vi "S4GUI.vi"(7 "Tab ObsEng":enum32{"Obs", "CCD modes", "Guider", "Eng"}(tab)) -> ()   [LabVIEW 2018] (continued)
            n3113 = call-dynamic "Write Object.vi"("error in (no error)"=w6663, "Object"=w6746, "Interface in"=w6666) -> ("error out"=w6664:errorcluster, "Interface out"=w6667:refnum<class "Interface.lvclass">)  [unwired: 7 in]
            n3114 = call-dynamic "Write Object.vi"("error in (no error)"=w6559, "Object"=w6746, "Interface in"=w6562) -> ("error out"=w6560:errorcluster, "Interface out"=w6563:refnum<class "Interface.lvclass">)  [unwired: 7 in]
            n3115 = call-dynamic "Write Object.vi"("error in (no error)"=w6618, "Object"=w6746, "Interface in"=w6615) -> ("error out"=w6617:errorcluster, "Interface out"=w6614:refnum<class "Interface.lvclass">)  [unwired: 7 in]
            n3116 = call-dynamic "Write Comments.vi"("error in (no error)"=w6664, "Comments"=w6745, "Interface in"=w6667) -> ("error out"=w6668:errorcluster, "Interface out"=w6669:refnum<class "Interface.lvclass">)  [unwired: 7 in]
            n3117 = call-dynamic "Write Comments.vi"("error in (no error)"=w6713, "Comments"=w6745, "Interface in"=w6717) -> ("error out"=w6718:errorcluster, "Interface out"=w6719:refnum<class "Interface.lvclass">)  [unwired: 7 in]
            n3118 = call-dynamic "Write Comments.vi"("error in (no error)"=w6560, "Comments"=w6745, "Interface in"=w6563) -> ("error out"=w6564:errorcluster, "Interface out"=w6565:refnum<class "Interface.lvclass">)  [unwired: 7 in]
            n3119 = call-dynamic "Write Comments.vi"("error in (no error)"=w6617, "Comments"=w6745, "Interface in"=w6614) -> ("error out"=w6613:errorcluster, "Interface out"=w6612:refnum<class "Interface.lvclass">)  [unwired: 7 in]
            n3120 = call-dynamic "Write Observer.vi"("error in (no error)"=w6668, "Observer"=w6744, "Interface in"=w6669) -> ("error out"=w6673:errorcluster, "Interface out"=w6672:refnum<class "Interface.lvclass">)  [unwired: 7 in]
            n3121 = call-dynamic "Write Observer.vi"("error in (no error)"=w6718, "Observer"=w6744, "Interface in"=w6719) -> ("error out"=w6723:errorcluster, "Interface out"=w6722:refnum<class "Interface.lvclass">)  [unwired: 7 in]
            n3122 = call-dynamic "Write Observer.vi"("error in (no error)"=w6564, "Observer"=w6744, "Interface in"=w6565) -> ("error out"=w6530:errorcluster, "Interface out"=w6531:refnum<class "Interface.lvclass">)  [unwired: 7 in]
            n3123 = call-dynamic "Write Observer.vi"("error in (no error)"=w6613, "Observer"=w6744, "Interface in"=w6612) -> ("error out"=w6608:errorcluster, "Interface out"=w6609:refnum<class "Interface.lvclass">)  [unwired: 7 in]
            n3124 = call-dynamic "Write Interface.vi"("error in (no error)"=w6723, "Interface.lvclass"=w6722, "Channel in"=w6714) -> ("error out"=w6706:errorcluster, "Channel out"=w6707:refnum<class "Channel.lvclass">)  [unwired: 7 in]
            n3125 = call-dynamic "Write Interface.vi"("error in (no error)"=w6608, "Interface.lvclass"=w6609, "Channel in"=w6621) -> ("error out"=w6585:errorcluster, "Channel out"=w6586:refnum<class "Channel.lvclass">)  [unwired: 7 in]
            n3126 = call-dynamic "Write Interface.vi"("error in (no error)"=w6673, "Interface.lvclass"=w6672, "Channel in"=w6659) -> ("error out"=w6637:errorcluster, "Channel out"=w6639:refnum<class "Channel.lvclass">)  [unwired: 7 in]
            n3127 = call-dynamic "Write Interface.vi"("error in (no error)"=w6530, "Interface.lvclass"=w6531, "Channel in"=w6532) -> ("error out"=w6535:errorcluster, "Channel out"=w6536:refnum<class "Channel.lvclass">)  [unwired: 7 in]
            n3128 = case shown="True" w6526 {
              tunnel: [w6874 w6896] -> w6727
              tunnel: [w6873 w6895] -> w6726
              tunnel: w6707 -> [w6874 w6894]
              tunnel: w6706 -> [w6873 w6893]
              frame False {
              }
              frame True {
                n3129 = call-dynamic "Read State Machine.vi"("error in (no error)"=w6893, "Device in"=w6894) -> ("error out"=w6890:errorcluster, "State Machine.lvclass"=w6891:refnum<class "State Machine.lvclass">, "Device out"=w6898:refnum<class "Channel.lvclass">)  [unwired: 7 in]
                n3130 = call-dynamic "Read ref StatesQueue.vi"("error in (no error)"=w6890, "State Machine in"=w6891) -> ("error out"=w6888:errorcluster, "ref StatesQueue"=w6889:refnum<queue>, "State Machine out"=w6885:refnum<class "State Machine.lvclass">)  [unwired: 7 in]
                n3131 = Flush Queue(queue=w6889, error in (no error)=w6888) -> (queue out=w6887:refnum<queue>, error out=w6883:errorcluster)  [unwired: 1 out]
                n3132 = Enqueue Element(queue=w6887, element=u32 300 ("State"), error in (no error)=w6883) -> (queue out=w6878:refnum<queue>, error out=w6876:errorcluster)  [unwired: 1 in, 1 out]
                n3133 = disable-structure shown="Enabled" {
                  disable-tunnel: w6878 -> [w6904 w6906]
                  disable-tunnel: [w6903 w6906] -> w6877
                  disable-tunnel: w6876 -> [w6902 w6905]
                  disable-tunnel: [w6901 w6905] -> w6875
                  frame Disabled {
                    n3134 = Enqueue Element(queue=w6904, element=u32 305 ("State"), error in (no error)=w6902) -> (queue out=w6903:refnum<queue>, error out=w6901:errorcluster)  [unwired: 1 in, 1 out]
                  }
                  frame Enabled {
                  }
                }
                n3135 = Enqueue Element(queue=w6877, element=u32 60 ("State"), error in (no error)=w6875) -> (queue out=w6886:refnum<queue>, error out=w6884:errorcluster)  [unwired: 1 in, 1 out]
                n3136 = call-dynamic "Write ref StatesQueue.vi"("error in (no error)"=w6884, "ref StatesQueue"=w6886, "State Machine in"=w6885) -> ("error out"=w6881:errorcluster, "State Machine out"=w6882:refnum<class "State Machine.lvclass">)  [unwired: 7 in]
                n3137 = call-dynamic "Write State.vi"("error in (no error)"=w6881, "State"=0, "State Machine in"=w6882) -> ("error out"=w6899:errorcluster, "State Machine out"=w6897:refnum<class "State Machine.lvclass">)  [unwired: 7 in]
                n3138 = call-dynamic "Write State Machine.vi"("error in (no error)"=w6899, "State Machine.lvclass"=w6897, "Device in"=w6898) -> ("error out"=w6895:errorcluster, "Device out"=w6896:refnum<class "Channel.lvclass">)  [unwired: 7 in]
              }
            }
            n3139 = case shown="True" w6527 {
              tunnel: w6639 -> [w6840 w6849]
              tunnel: [w6840 w6847] -> w6638
              tunnel: w6637 -> [w6839 w6846]
              tunnel: [w6839 w6845] -> w6636
              frame False {
              }
              frame True {
                n3140 = call-dynamic "Read State Machine.vi"("error in (no error)"=w6846, "Device in"=w6849) -> ("error out"=w6861:errorcluster, "State Machine.lvclass"=w6862:refnum<class "State Machine.lvclass">, "Device out"=w6848:refnum<class "Channel.lvclass">)  [unwired: 7 in]
                n3141 = call-dynamic "Read ref StatesQueue.vi"("error in (no error)"=w6861, "State Machine in"=w6862) -> ("error out"=w6859:errorcluster, "ref StatesQueue"=w6860:refnum<queue>, "State Machine out"=w6856:refnum<class "State Machine.lvclass">)  [unwired: 7 in]
                n3142 = Flush Queue(queue=w6860, error in (no error)=w6859) -> (queue out=w6858:refnum<queue>, error out=w6854:errorcluster)  [unwired: 1 out]
                n3143 = Enqueue Element(queue=w6858, element=u32 300 ("State"), error in (no error)=w6854) -> (queue out=w6844:refnum<queue>, error out=w6842:errorcluster)  [unwired: 1 in, 1 out]
                n3144 = disable-structure shown="Enabled" {
                  disable-tunnel: w6844 -> [w6869 w6872]
                  disable-tunnel: [w6868 w6872] -> w6843
                  disable-tunnel: w6842 -> [w6867 w6871]
                  disable-tunnel: [w6866 w6871] -> w6841
                  frame Disabled {
                    n3145 = Enqueue Element(queue=w6869, element=u32 305 ("State"), error in (no error)=w6867) -> (queue out=w6868:refnum<queue>, error out=w6866:errorcluster)  [unwired: 1 in, 1 out]
                  }
                  frame Enabled {
                  }
                }
                n3146 = Enqueue Element(queue=w6843, element=u32 60 ("State"), error in (no error)=w6841) -> (queue out=w6857:refnum<queue>, error out=w6855:errorcluster)  [unwired: 1 in, 1 out]
                n3147 = call-dynamic "Write ref StatesQueue.vi"("error in (no error)"=w6855, "ref StatesQueue"=w6857, "State Machine in"=w6856) -> ("error out"=w6852:errorcluster, "State Machine out"=w6853:refnum<class "State Machine.lvclass">)  [unwired: 7 in]
                n3148 = call-dynamic "Write State.vi"("error in (no error)"=w6852, "State"=0, "State Machine in"=w6853) -> ("error out"=w6865:errorcluster, "State Machine out"=w6864:refnum<class "State Machine.lvclass">)  [unwired: 7 in]
                n3149 = call-dynamic "Write State Machine.vi"("error in (no error)"=w6865, "State Machine.lvclass"=w6864, "Device in"=w6848) -> ("error out"=w6845:errorcluster, "Device out"=w6847:refnum<class "Channel.lvclass">)  [unwired: 7 in]
              }
            }
            n3150 = case shown="True" w6528 {
              tunnel: w6586 -> [w6806 w6814]
              tunnel: w6585 -> [w6805 w6813]
              tunnel: [w6805 w6812] -> w6584
              tunnel: [w6806 w6811] -> w6583
              frame False {
              }
              frame True {
                n3151 = call-dynamic "Read State Machine.vi"("error in (no error)"=w6813, "Device in"=w6814) -> ("error out"=w6827:errorcluster, "State Machine.lvclass"=w6828:refnum<class "State Machine.lvclass">, "Device out"=w6815:refnum<class "Channel.lvclass">)  [unwired: 7 in]
                n3152 = call-dynamic "Read ref StatesQueue.vi"("error in (no error)"=w6827, "State Machine in"=w6828) -> ("error out"=w6825:errorcluster, "ref StatesQueue"=w6826:refnum<queue>, "State Machine out"=w6822:refnum<class "State Machine.lvclass">)  [unwired: 7 in]
                n3153 = Flush Queue(queue=w6826, error in (no error)=w6825) -> (queue out=w6824:refnum<queue>, error out=w6820:errorcluster)  [unwired: 1 out]
                n3154 = Enqueue Element(queue=w6824, element=u32 300 ("State"), error in (no error)=w6820) -> (queue out=w6810:refnum<queue>, error out=w6808:errorcluster)  [unwired: 1 in, 1 out]
                n3155 = disable-structure shown="Enabled" {
                  disable-tunnel: w6810 -> [w6835 w6838]
                  disable-tunnel: [w6834 w6838] -> w6809
                  disable-tunnel: w6808 -> [w6833 w6837]
                  disable-tunnel: [w6832 w6837] -> w6807
                  frame Disabled {
                    n3156 = Enqueue Element(queue=w6835, element=u32 305 ("State"), error in (no error)=w6833) -> (queue out=w6834:refnum<queue>, error out=w6832:errorcluster)  [unwired: 1 in, 1 out]
                  }
                  frame Enabled {
                  }
                }
                n3157 = Enqueue Element(queue=w6809, element=u32 60 ("State"), error in (no error)=w6807) -> (queue out=w6823:refnum<queue>, error out=w6821:errorcluster)  [unwired: 1 in, 1 out]
                n3158 = call-dynamic "Write ref StatesQueue.vi"("error in (no error)"=w6821, "ref StatesQueue"=w6823, "State Machine in"=w6822) -> ("error out"=w6818:errorcluster, "State Machine out"=w6819:refnum<class "State Machine.lvclass">)  [unwired: 7 in]
                n3159 = call-dynamic "Write State.vi"("error in (no error)"=w6818, "State"=0, "State Machine in"=w6819) -> ("error out"=w6831:errorcluster, "State Machine out"=w6830:refnum<class "State Machine.lvclass">)  [unwired: 7 in]
                n3160 = call-dynamic "Write State Machine.vi"("error in (no error)"=w6831, "State Machine.lvclass"=w6830, "Device in"=w6815) -> ("error out"=w6812:errorcluster, "Device out"=w6811:refnum<class "Channel.lvclass">)  [unwired: 7 in]
              }
            }
            n3161 = case shown="True" w6529 {
              tunnel: w6536 -> [w6772 w6784]
              tunnel: w6535 -> [w6771 w6783]
              tunnel: [w6771 w6782] -> w6534
              tunnel: [w6772 w6781] -> w6533
              frame False {
              }
              frame True {
                n3162 = call-dynamic "Read State Machine.vi"("error in (no error)"=w6783, "Device in"=w6784) -> ("error out"=w6795:errorcluster, "State Machine.lvclass"=w6780:refnum<class "State Machine.lvclass">, "Device out"=w6785:refnum<class "Channel.lvclass">)  [unwired: 7 in]
                n3163 = call-dynamic "Read ref StatesQueue.vi"("error in (no error)"=w6795, "State Machine in"=w6780) -> ("error out"=w6793:errorcluster, "ref StatesQueue"=w6794:refnum<queue>, "State Machine out"=w6779:refnum<class "State Machine.lvclass">)  [unwired: 7 in]
                n3164 = Flush Queue(queue=w6794, error in (no error)=w6793) -> (queue out=w6792:refnum<queue>, error out=w6789:errorcluster)  [unwired: 1 out]
                n3165 = Enqueue Element(queue=w6792, element=u32 300 ("State"), error in (no error)=w6789) -> (queue out=w6776:refnum<queue>, error out=w6775:errorcluster)  [unwired: 1 in, 1 out]
                n3166 = disable-structure shown="Enabled" {
                  disable-tunnel: w6776 -> [w6801 w6804]
                  disable-tunnel: w6775 -> [w6800 w6803]
                  disable-tunnel: [w6799 w6804] -> w6774
                  disable-tunnel: [w6798 w6803] -> w6773
                  frame Disabled {
                    n3167 = Enqueue Element(queue=w6801, element=u32 305 ("State"), error in (no error)=w6800) -> (queue out=w6799:refnum<queue>, error out=w6798:errorcluster)  [unwired: 1 in, 1 out]
                  }
                  frame Enabled {
                  }
                }
                n3168 = Enqueue Element(queue=w6774, element=u32 60 ("State"), error in (no error)=w6773) -> (queue out=w6791:refnum<queue>, error out=w6790:errorcluster)  [unwired: 1 in, 1 out]
                n3169 = call-dynamic "Write ref StatesQueue.vi"("error in (no error)"=w6790, "ref StatesQueue"=w6791, "State Machine in"=w6779) -> ("error out"=w6788:errorcluster, "State Machine out"=w6778:refnum<class "State Machine.lvclass">)  [unwired: 7 in]
                n3170 = call-dynamic "Write State.vi"("error in (no error)"=w6788, "State"=0, "State Machine in"=w6778) -> ("error out"=w6797:errorcluster, "State Machine out"=w6777:refnum<class "State Machine.lvclass">)  [unwired: 7 in]
                n3171 = call-dynamic "Write State Machine.vi"("error in (no error)"=w6797, "State Machine.lvclass"=w6777, "Device in"=w6785) -> ("error out"=w6782:errorcluster, "Device out"=w6781:refnum<class "Channel.lvclass">)  [unwired: 7 in]
              }
            }
            n3172 = call-dynamic "Write Channel.vi"("error in (no error)"=w6726, "Channel.lvclass"=w6727, "Acquisition in"=w6741) -> ("error out"=w6769:errorcluster, "Acquisition out"=w6770:refnum<class "Acquisition.lvclass">)  [unwired: 7 in]
            n3173 = call-dynamic "Write Channel.vi"("error in (no error)"=w6636, "Channel.lvclass"=w6638, "Acquisition in"=w6675) -> ("error out"=w6767:errorcluster, "Acquisition out"=w6768:refnum<class "Acquisition.lvclass">)  [unwired: 7 in]
            n3174 = call-dynamic "Write Channel.vi"("error in (no error)"=w6584, "Channel.lvclass"=w6583, "Acquisition in"=w6622) -> ("error out"=w6765:errorcluster, "Acquisition out"=w6766:refnum<class "Acquisition.lvclass">)  [unwired: 7 in]
            n3175 = call-dynamic "Write Channel.vi"("error in (no error)"=w6534, "Channel.lvclass"=w6533, "Acquisition in"=w6582) -> ("error out"=w6763:errorcluster, "Acquisition out"=w6764:refnum<class "Acquisition.lvclass">)  [unwired: 7 in]
          }
        }
        n3176 = call-dynamic "Write AcquisitionA.vi"("error in (no error)"=w5658, "Acquisition.lvclass"=w5659, "S4ACS_GUI in"=w5660) -> ("error out"=w5650:errorcluster, "S4ACS_GUI out"=w5654:refnum<class "S4GUI.lvclass">)  [unwired: 7 in]
        n3177 = call "Write AcquisitionB.vi"("error in (no error)"=w5655, "Acquisition.lvclass"=w5656, "S4ACS_GUI in"=w5654) -> ("error out"=w5649:errorcluster, "S4ACS_GUI out"=w5653:refnum<class "S4GUI.lvclass">)  [unwired: 7 in]
        n3178 = call-dynamic "Write AcquisitionC.vi"("error in (no error)"=w5644, "Acquisition.lvclass"=w5645, "S4ACS_GUI in"=w5653) -> ("error out"=w5648:errorcluster, "S4ACS_GUI out"=w5652:refnum<class "S4GUI.lvclass">)  [unwired: 7 in]
        n3179 = call-dynamic "Write AcquisitionD.vi"("error in (no error)"=w5642, "Acquisition.lvclass"=w5643, "S4ACS_GUI in"=w5652) -> ("error out"=w5647:errorcluster, "S4ACS_GUI out"=w5651:refnum<class "S4GUI.lvclass">)  [unwired: 7 in]
        n3180 = Merge Errors(w5650, w5649, w5648, w5647) -> (w5646:errorcluster)
        n3181 = call "Write cfg file.vi"("error in (no error)"=w5646, "cfg file"="lastsaved.cfg", "S4ACS_GUI in"=w5651) -> ("error out"=w5602:errorcluster, "S4ACS_GUI out"=w5603:refnum<class "S4GUI.lvclass">)  [unwired: 7 in]
        n3182 = disable-structure shown="Enabled" {
          disable-tunnel: w5603 -> [w5664 w5699]
          disable-tunnel: w5602 -> [w5663 w5698]
          disable-tunnel: [w5662 w5699] -> w5601
          disable-tunnel: [w5661 w5698] -> w5600
          frame Disabled {
            # "Este código passou para o evento \"Timeout\" (executa sempre)"
            # "1a vez FOTOM (F)"
            # "1a vez POLAR (F)"
            n3183 = call "Read Instrument.lvclass.vi"("error in (no error)"=w5663, "S4ACS_GUI in"=w5664) -> ("error out"=w5666:errorcluster, "Instrument.lvclass"=w5667:refnum<class "Instrument.lvclass">, "S4ACS_GUI out"=w5662:refnum<class "S4GUI.lvclass">)  [unwired: 7 in]
            n3184 = call-dynamic "Read mode.vi"("error in (no error)"=w5666, "Instrument in"=w5667) -> ("error out"=w5661:errorcluster, "mode"=w5665:bool)  [unwired: 7 in, 1 out]
            n3185 = while {
              tunnel: w5665 -> [w5672]
              shift-right: [w5668] -> _
              shift-left: _ -> [w5671]
              shift-right: [w5669] -> _
              shift-left: _ -> [w5670]
              stop <- TRUE stop-if-true
              # "Valores default para procedimento\nde ajuste de foco do telescópio"
              n3186 = case shown="True" w5672 {
                tunnel: w5671 -> [w5674 w5689]
                tunnel: [w5675 w5688] -> w5668
                tunnel: w5670 -> [w5677 w5687]
                tunnel: [w5676 w5686] -> w5669
                frame True {
                  # "polarimetria"
                  n3187 = case shown="False" w5677 {
                    selector: w5677 -> [w5681 w5685]
                    tunnel: [w5680 w5685] -> w5676
                    tunnel: [FALSE FALSE] -> w5675
                    tunnel: w5674 -> [_ _]
                    frame False {
                      w5678 = 12900
                      n3188 = local write "Start focus"(w5678) -> ()
                      n3189 = local write "Target focus"(w5678) -> ()
                      n3190 = local write "Step focus"(80) -> ()
                      n3191 = local write "#steps"(11) -> ()
                      n3192 = Not(x=w5681) -> (.not. x?=w5680:bool)
                    }
                    frame True {
                    }
                  }
                }
                frame False {
                  # "fotometria"
                  n3193 = case shown="False" w5689 {
                    selector: w5689 -> [w5692 w5697]
                    tunnel: [w5691 w5697] -> w5688
                    tunnel: w5687 -> [_ _]
                    tunnel: [FALSE FALSE] -> w5686
                    frame False {
                      w5690 = 13400
                      n3194 = local write "Start focus"(w5690) -> ()
                      n3195 = local write "Step focus"(100) -> ()
                      n3196 = local write "Target focus"(w5690) -> ()
                      n3197 = local write "#steps"(11) -> ()
                      n3198 = Not(x=w5692) -> (.not. x?=w5691:bool)
                    }
                    frame True {
                    }
                  }
                }
              }
            }
          }
          frame Enabled {
          }
        }
      }
      event "set keywords", "set Observer": Value Change {
        # "Observer: max len = 54\nProject ID: max len = 15\nObject: max len = 30"
        # "SET suffix e publica os outros campos da aba selecionada."
        n3199 = event-data() -> ()  [unwired: 1 in, 1 out]
        n3200 = local read "Tab Acq Type"() -> (w6968:T1)
        n3201 = case shown="\"DARK\"" w6968 {
          tunnel: ["OBJECT" "FLAT" "FLAT" "DARK" "ZERO" "FOCUS"] -> w7084
          tunnel: [w7190 w7194 w7198 w7202 w7206 w7210] -> w6967
          tunnel: [w7189 w7193 w7197 w7201 w7205 w7209] -> w7081
          tunnel: [w7188 w7192 w7196 w7200 w7204 w7208] -> w7080
          frame "OBJECT", Default {
            n3202 = local read "OBJECT Comments"() -> (w7188:string)
            n3203 = local read "Object_obj"() -> (w7190:string)
            n3204 = local read "object suffix"() -> (w7189:string)
          }
          frame "DFLAT" {
            n3205 = local read "DFLAT Comments"() -> (w7192:string)
            n3206 = local read "Object_dflat"() -> (w7194:string)
            n3207 = local read "dflat suffix"() -> (w7193:string)
          }
          frame "SFLAT" {
            n3208 = local read "SFLAT Comments"() -> (w7196:string)
            n3209 = local read "Object_sflat"() -> (w7198:string)
            n3210 = local read "sflat suffix"() -> (w7197:string)
          }
          frame "DARK" {
            n3211 = local read "DARK Comments"() -> (w7200:string)
            n3212 = local read "Object_dark"() -> (w7202:string)
            n3213 = local read "dark suffix"() -> (w7201:string)
          }
          frame "ZERO" {
            n3214 = local read "ZERO Comments"() -> (w7204:string)
            n3215 = local read "Object_zero"() -> (w7206:string)
            n3216 = local read "zero suffix"() -> (w7205:string)
          }
          frame "FOCUS" {
            n3217 = local read "FOCUS Comments"() -> (w7208:string)
            n3218 = local read "Object_focus"() -> (w7210:string)
            n3219 = local read "focus suffix"() -> (w7209:string)
          }
        }
        n3220 = String Subset(string=w6961, length (rest)=15 ("length (rest)")) -> (substring=w6959:string)  [unwired: 1 in]
        n3221 = String Subset(string=w6963, length (rest)=54 ("length (rest)")) -> (substring=w6960:string)  [unwired: 1 in]
        n3222 = local write "Observer"(w6960) -> ()
        n3223 = local write "Project ID"(w6959) -> ()
        n3224 = String Subset(string=w6967, length (rest)=30 ("length (rest)")) -> (substring=w6965:string)  [unwired: 1 in]
        n3225 = case shown="\"OBJECT\", Default" w6968 {
          tunnel: w6965 -> [w7134 w7135 w7136 w7137 w7138 w7139]
          frame "OBJECT", Default {
            n3226 = local write "Object_obj"(w7134) -> ()
          }
          frame "DFLAT" {
            n3227 = local write "Object_dflat"(w7135) -> ()
          }
          frame "SFLAT" {
            n3228 = local write "Object_sflat"(w7136) -> ()
          }
          frame "DARK" {
            n3229 = local write "Object_dark"(w7137) -> ()
          }
          frame "ZERO" {
            n3230 = local write "Object_zero"(w7138) -> ()
          }
          frame "FOCUS" {
            n3231 = local write "Object_focus"(w7139) -> ()
          }
        }
        n3232 = call-dynamic "Write User Event.vi"("error in (no error)"=w7075, "User Event"="SET KEYWORDS CLICKED (Obsever, ProjectID, Object, Comments) ", "S4GUI in"=w7076) -> ("error out"=w7073:errorcluster, "S4GUI out"=w7074:refnum<class "S4GUI.lvclass">)  [unwired: 7 in]
        n3233 = call-dynamic "Read Publisher.lvclass.vi"("error in (no error)"=w7073, "S4GUI in"=w7074) -> ("error out"=w7094:errorcluster, "Publisher.lvclass"=w7090:refnum<class "Publisher.lvclass">, "S4GUI out"=w7095:refnum<class "S4GUI.lvclass">)  [unwired: 7 in]
        n3234 = call-dynamic "Write object.vi"("error in (no error)"=w7094, "object"=w6965, "Publisher in"=w7090) -> ("error out"=w7093:errorcluster, "Publisher out"=w7089:refnum<class "Publisher.lvclass">)  [unwired: 7 in]
        n3235 = call-dynamic "Write obstype.vi"("error in (no error)"=w7093, "obstype"=w7084, "Publisher in"=w7089) -> ("error out"=w7092:errorcluster, "Publisher out"=w7088:refnum<class "Publisher.lvclass">)  [unwired: 7 in]
        n3236 = call-dynamic "Write observer.vi"("error in (no error)"=w7092, "observer"=w6960, "Publisher in"=w7088) -> ("error out"=w7091:errorcluster, "Publisher out"=w7087:refnum<class "Publisher.lvclass">)  [unwired: 7 in]
        n3237 = call-dynamic "Write projid.vi"("error in (no error)"=w7091, "projid"=w6959, "Publisher in"=w7087) -> ("error out"=w7079:errorcluster, "Publisher out"=w7078:refnum<class "Publisher.lvclass">)  [unwired: 7 in]
        n3238 = call-dynamic "Write comments.vi"("error in (no error)"=w7079, "comments"=w7080, "Publisher in"=w7078) -> ("error out"=w7083:errorcluster, "Publisher out"=w7082:refnum<class "Publisher.lvclass">)  [unwired: 7 in]
        n3239 = call-dynamic "Write Publisher.lvclass.vi"("error in (no error)"=w7083, "Publisher.lvclass"=w7082, "S4GUI in"=w7095) -> ("error out"=w7085:errorcluster, "S4GUI out"=w7086:refnum<class "S4GUI.lvclass">)  [unwired: 7 in]
        n3240 = call-dynamic "Read AcquisitionC.vi"("error in (no error)"=w7085, "S4ACS_GUI in"=w7086) -> ("error out"=w7107:errorcluster, "Acquisition.lvclass"=w7108:refnum<class "Acquisition.lvclass">)  [unwired: 7 in, 1 out]
        n3241 = call-dynamic "Read AcquisitionA.vi"("error in (no error)"=w7085, "S4ACS_GUI in"=w7086) -> ("error out"=w7111:errorcluster, "Acquisition.lvclass"=w7112:refnum<class "Acquisition.lvclass">, "S4ACS_GUI out"=w7133:refnum<class "S4GUI.lvclass">)  [unwired: 7 in]
        n3242 = call "Read AcquisitionB.vi"("error in (no error)"=w7085, "S4ACS_GUI in"=w7086) -> ("error out"=w7109:errorcluster, "Acquisition.lvclass"=w7110:refnum<class "Acquisition.lvclass">)  [unwired: 7 in, 1 out]
        n3243 = call-dynamic "Read AcquisitionD.vi"("error in (no error)"=w7085, "S4ACS_GUI in"=w7086) -> ("error out"=w7105:errorcluster, "Acquisition.lvclass"=w7106:refnum<class "Acquisition.lvclass">)  [unwired: 7 in, 1 out]
        n3244 = call-dynamic "Read enabled.vi"("error in (no error)"=w7107, "Server in"=w7108) -> ("error out"=w7098:errorcluster, "enabled"=w6995:bool, "Server out"=w7099:refnum<class "Acquisition.lvclass">)  [unwired: 7 in]
        n3245 = call-dynamic "Read enabled.vi"("error in (no error)"=w7105, "Server in"=w7106) -> ("error out"=w7096:errorcluster, "enabled"=w6969:bool, "Server out"=w7097:refnum<class "Acquisition.lvclass">)  [unwired: 7 in]
        n3246 = call-dynamic "Read enabled.vi"("error in (no error)"=w7109, "Server in"=w7110) -> ("error out"=w7100:errorcluster, "enabled"=w7021:bool, "Server out"=w7101:refnum<class "Acquisition.lvclass">)  [unwired: 7 in]
        n3247 = call-dynamic "Read enabled.vi"("error in (no error)"=w7111, "Server in"=w7112) -> ("error out"=w7102:errorcluster, "enabled"=w7047:bool, "Server out"=w7103:refnum<class "Acquisition.lvclass">)  [unwired: 7 in]
        n3248 = call-dynamic "Read Channel.vi"("error in (no error)"=w7100, "Acquisition in"=w7101) -> ("error out"=w7026:errorcluster, "Channel.lvclass"=w7027:refnum<class "Channel.lvclass">, "Acquisition out"=w7044:refnum<class "Acquisition.lvclass">)  [unwired: 7 in]
        n3249 = call-dynamic "Read Channel.vi"("error in (no error)"=w7096, "Acquisition in"=w7097) -> ("error out"=w6974:errorcluster, "Channel.lvclass"=w6975:refnum<class "Channel.lvclass">, "Acquisition out"=w6994:refnum<class "Acquisition.lvclass">)  [unwired: 7 in]
        n3250 = call-dynamic "Read Channel.vi"("error in (no error)"=w7098, "Acquisition in"=w7099) -> ("error out"=w7000:errorcluster, "Channel.lvclass"=w7001:refnum<class "Channel.lvclass">, "Acquisition out"=w7018:refnum<class "Acquisition.lvclass">)  [unwired: 7 in]
        n3251 = call-dynamic "Read Channel.vi"("error in (no error)"=w7102, "Acquisition in"=w7103) -> ("error out"=w7052:errorcluster, "Channel.lvclass"=w7053:refnum<class "Channel.lvclass">, "Acquisition out"=w7072:refnum<class "Acquisition.lvclass">)  [unwired: 7 in]
        n3252 = To Lower Case(string=w7081) -> (all lower case string=w7104:string)
        n3253 = local read "Filter2"() -> (w7028:u8)
        n3254 = local read "Filter4"() -> (w6976:u8)
        n3255 = local read "Filter3"() -> (w7002:u8)
        n3256 = local read "Filter1"() -> (w7056:u8)
        n3257 = call-dynamic "Write Filter.vi"("error in (no error)"=w6974, "Filter"=w6976, "Channel in"=w6975) -> ("error out"=w6991:errorcluster, "Channel out"=w6980:refnum<class "Channel.lvclass">)  [unwired: 7 in]
        n3258 = call-dynamic "Write Filter.vi"("error in (no error)"=w7026, "Filter"=w7028, "Channel in"=w7027) -> ("error out"=w7043:errorcluster, "Channel out"=w7032:refnum<class "Channel.lvclass">)  [unwired: 7 in]
        n3259 = call-dynamic "Write Filter.vi"("error in (no error)"=w7000, "Filter"=w7002, "Channel in"=w7001) -> ("error out"=w7005:errorcluster, "Channel out"=w7016:refnum<class "Channel.lvclass">)  [unwired: 7 in]
        n3260 = call-dynamic "Write Filter.vi"("error in (no error)"=w7052, "Filter"=w7056, "Channel in"=w7053) -> ("error out"=w7069:errorcluster, "Channel out"=w7068:refnum<class "Channel.lvclass">)  [unwired: 7 in]
        n3261 = call-dynamic "Read Interface.vi"("error in (no error)"=w6991, "Channel in"=w6980) -> ("error out"=w6990:errorcluster, "Interface.lvclass"=w6989:refnum<class "Interface.lvclass">, "Channel out"=w6979:refnum<class "Channel.lvclass">)  [unwired: 7 in]
        n3262 = call-dynamic "Read Interface.vi"("error in (no error)"=w7043, "Channel in"=w7032) -> ("error out"=w7042:errorcluster, "Interface.lvclass"=w7041:refnum<class "Interface.lvclass">, "Channel out"=w7031:refnum<class "Channel.lvclass">)  [unwired: 7 in]
        n3263 = call-dynamic "Read Interface.vi"("error in (no error)"=w7005, "Channel in"=w7016) -> ("error out"=w7006:errorcluster, "Interface.lvclass"=w7007:refnum<class "Interface.lvclass">, "Channel out"=w7017:refnum<class "Channel.lvclass">)  [unwired: 7 in]
        n3264 = call-dynamic "Read Interface.vi"("error in (no error)"=w7069, "Channel in"=w7068) -> ("error out"=w7067:errorcluster, "Interface.lvclass"=w7066:refnum<class "Interface.lvclass">, "Channel out"=w7060:refnum<class "Channel.lvclass">)  [unwired: 7 in]
        n3265 = call-dynamic "Write Suffix.vi"("error in (no error)"=w7067, "Suffix"=w7104, "Interface in"=w7066) -> ("error out"=w7057:errorcluster, "Interface out"=w7061:refnum<class "Interface.lvclass">)  [unwired: 7 in]
        n3266 = call-dynamic "Write Suffix.vi"("error in (no error)"=w6990, "Suffix"=w7104, "Interface in"=w6989) -> ("error out"=w6981:errorcluster, "Interface out"=w6984:refnum<class "Interface.lvclass">)  [unwired: 7 in]
        n3267 = call-dynamic "Write Suffix.vi"("error in (no error)"=w7042, "Suffix"=w7104, "Interface in"=w7041) -> ("error out"=w7033:errorcluster, "Interface out"=w7036:refnum<class "Interface.lvclass">)  [unwired: 7 in]
        n3268 = call-dynamic "Write Suffix.vi"("error in (no error)"=w7006, "Suffix"=w7104, "Interface in"=w7007) -> ("error out"=w7015:errorcluster, "Interface out"=w7012:refnum<class "Interface.lvclass">)  [unwired: 7 in]
        n3269 = call-dynamic "Write ObsType.vi"("error in (no error)"=w7057, "ObsType"=w7084, "Interface in"=w7061) -> ("error out"=w7058:errorcluster, "Interface out"=w7062:refnum<class "Interface.lvclass">)  [unwired: 7 in]
        n3270 = call-dynamic "Write ObsType.vi"("error in (no error)"=w6981, "ObsType"=w7084, "Interface in"=w6984) -> ("error out"=w6982:errorcluster, "Interface out"=w6985:refnum<class "Interface.lvclass">)  [unwired: 7 in]
        n3271 = call-dynamic "Write ObsType.vi"("error in (no error)"=w7033, "ObsType"=w7084, "Interface in"=w7036) -> ("error out"=w7034:errorcluster, "Interface out"=w7037:refnum<class "Interface.lvclass">)  [unwired: 7 in]
        n3272 = call-dynamic "Write ObsType.vi"("error in (no error)"=w7015, "ObsType"=w7084, "Interface in"=w7012) -> ("error out"=w7014:errorcluster, "Interface out"=w7011:refnum<class "Interface.lvclass">)  [unwired: 7 in]
        n3273 = call-dynamic "Write Object.vi"("error in (no error)"=w7058, "Object"=w6965, "Interface in"=w7062) -> ("error out"=w7059:errorcluster, "Interface out"=w7063:refnum<class "Interface.lvclass">)  [unwired: 7 in]
        n3274 = call-dynamic "Write Object.vi"("error in (no error)"=w7034, "Object"=w6965, "Interface in"=w7037) -> ("error out"=w7035:errorcluster, "Interface out"=w7038:refnum<class "Interface.lvclass">)  [unwired: 7 in]
        n3275 = call-dynamic "Write Object.vi"("error in (no error)"=w6982, "Object"=w6967, "Interface in"=w6985) -> ("error out"=w6983:errorcluster, "Interface out"=w6986:refnum<class "Interface.lvclass">)  [unwired: 7 in]
        n3276 = call-dynamic "Write Object.vi"("error in (no error)"=w7014, "Object"=w6965, "Interface in"=w7011) -> ("error out"=w7013:errorcluster, "Interface out"=w7010:refnum<class "Interface.lvclass">)  [unwired: 7 in]
        n3277 = call-dynamic "Write Comments.vi"("error in (no error)"=w6983, "Comments"=w7080, "Interface in"=w6986) -> ("error out"=w6987:errorcluster, "Interface out"=w6988:refnum<class "Interface.lvclass">)  [unwired: 7 in]
        n3278 = call-dynamic "Write Comments.vi"("error in (no error)"=w7035, "Comments"=w7080, "Interface in"=w7038) -> ("error out"=w7039:errorcluster, "Interface out"=w7040:refnum<class "Interface.lvclass">)  [unwired: 7 in]
        n3279 = call-dynamic "Write Comments.vi"("error in (no error)"=w7013, "Comments"=w7080, "Interface in"=w7010) -> ("error out"=w7009:errorcluster, "Interface out"=w7008:refnum<class "Interface.lvclass">)  [unwired: 7 in]
        n3280 = call-dynamic "Write Comments.vi"("error in (no error)"=w7059, "Comments"=w7080, "Interface in"=w7063) -> ("error out"=w7064:errorcluster, "Interface out"=w7065:refnum<class "Interface.lvclass">)  [unwired: 7 in]
        n3281 = call-dynamic "Write Observer.vi"("error in (no error)"=w6987, "Observer"=w6960, "Interface in"=w6988) -> ("error out"=w6973:errorcluster, "Interface out"=w6972:refnum<class "Interface.lvclass">)  [unwired: 7 in]
        n3282 = call-dynamic "Write Observer.vi"("error in (no error)"=w7064, "Observer"=w6960, "Interface in"=w7065) -> ("error out"=w7050:errorcluster, "Interface out"=w7051:refnum<class "Interface.lvclass">)  [unwired: 7 in]
        n3283 = call-dynamic "Write Observer.vi"("error in (no error)"=w7039, "Observer"=w6960, "Interface in"=w7040) -> ("error out"=w7025:errorcluster, "Interface out"=w7024:refnum<class "Interface.lvclass">)  [unwired: 7 in]
        n3284 = call-dynamic "Write Observer.vi"("error in (no error)"=w7009, "Observer"=w6960, "Interface in"=w7008) -> ("error out"=w6999:errorcluster, "Interface out"=w6998:refnum<class "Interface.lvclass">)  [unwired: 7 in]
        n3285 = call-dynamic "Write Project ID.vi"("error in (no error)"=w6999, "Project ID"=w6959, "Interface in"=w6998) -> ("error out"=w6996:errorcluster, "Interface out"=w6997:refnum<class "Interface.lvclass">)  [unwired: 7 in]
        n3286 = call-dynamic "Write Project ID.vi"("error in (no error)"=w7025, "Project ID"=w6959, "Interface in"=w7024) -> ("error out"=w7022:errorcluster, "Interface out"=w7023:refnum<class "Interface.lvclass">)  [unwired: 7 in]
        n3287 = call-dynamic "Write Project ID.vi"("error in (no error)"=w6973, "Project ID"=w6959, "Interface in"=w6972) -> ("error out"=w6970:errorcluster, "Interface out"=w6971:refnum<class "Interface.lvclass">)  [unwired: 7 in]
        n3288 = call-dynamic "Write Project ID.vi"("error in (no error)"=w7050, "Project ID"=w6959, "Interface in"=w7051) -> ("error out"=w7048:errorcluster, "Interface out"=w7049:refnum<class "Interface.lvclass">)  [unwired: 7 in]
        n3289 = call-dynamic "Write Interface.vi"("error in (no error)"=w7022, "Interface.lvclass"=w7023, "Channel in"=w7031) -> ("error out"=w7029:errorcluster, "Channel out"=w7030:refnum<class "Channel.lvclass">)  [unwired: 7 in]
        n3290 = call-dynamic "Write Interface.vi"("error in (no error)"=w7048, "Interface.lvclass"=w7049, "Channel in"=w7060) -> ("error out"=w7054:errorcluster, "Channel out"=w7055:refnum<class "Channel.lvclass">)  [unwired: 7 in]
        n3291 = call-dynamic "Write Interface.vi"("error in (no error)"=w6996, "Interface.lvclass"=w6997, "Channel in"=w7017) -> ("error out"=w7003:errorcluster, "Channel out"=w7004:refnum<class "Channel.lvclass">)  [unwired: 7 in]
        n3292 = call-dynamic "Write Interface.vi"("error in (no error)"=w6970, "Interface.lvclass"=w6971, "Channel in"=w6979) -> ("error out"=w6977:errorcluster, "Channel out"=w6978:refnum<class "Channel.lvclass">)  [unwired: 7 in]
        n3293 = case shown="True" w7021 {
          tunnel: [w7164 w7175] -> w7046
          tunnel: [w7165 w7174] -> w7045
          tunnel: w7030 -> [w7165 w7167]
          tunnel: w7029 -> [w7164 w7166]
          frame False {
          }
          frame True {
            # "command SET SUFFIX"
            n3294 = call-dynamic "Read State Machine.vi"("error in (no error)"=w7166, "Device in"=w7167) -> ("error out"=w7168:errorcluster, "State Machine.lvclass"=w7172:refnum<class "State Machine.lvclass">, "Device out"=w7171:refnum<class "Channel.lvclass">)  [unwired: 7 in]
            n3295 = call-dynamic "Write State.vi"("error in (no error)"=w7168, "State"=300, "State Machine in"=w7172) -> ("error out"=w7169:errorcluster, "State Machine out"=w7173:refnum<class "State Machine.lvclass">)  [unwired: 7 in]
            n3296 = call-dynamic "Write State Machine.vi"("error in (no error)"=w7169, "State Machine.lvclass"=w7173, "Device in"=w7171) -> ("error out"=w7175:errorcluster, "Device out"=w7174:refnum<class "Channel.lvclass">)  [unwired: 7 in]
          }
        }
        n3297 = case shown="True" w7047 {
          tunnel: [w7177 w7181] -> w7071
          tunnel: [w7176 w7180] -> w7070
          tunnel: w7055 -> [w7177 w7179]
          tunnel: w7054 -> [w7176 w7178]
          frame False {
          }
          frame True {
            # "command SET SUFFIX"
            n3298 = call-dynamic "Read State Machine.vi"("error in (no error)"=w7178, "Device in"=w7179) -> ("error out"=w7187:errorcluster, "State Machine.lvclass"=w7183:refnum<class "State Machine.lvclass">, "Device out"=w7184:refnum<class "Channel.lvclass">)  [unwired: 7 in]
            n3299 = call-dynamic "Write State.vi"("error in (no error)"=w7187, "State"=300, "State Machine in"=w7183) -> ("error out"=w7186:errorcluster, "State Machine out"=w7182:refnum<class "State Machine.lvclass">)  [unwired: 7 in]
            n3300 = call-dynamic "Write State Machine.vi"("error in (no error)"=w7186, "State Machine.lvclass"=w7182, "Device in"=w7184) -> ("error out"=w7180:errorcluster, "Device out"=w7181:refnum<class "Channel.lvclass">)  [unwired: 7 in]
          }
        }
        n3301 = case shown="True" w6995 {
          tunnel: [w7152 w7163] -> w7020
          tunnel: [w7153 w7162] -> w7019
          tunnel: w7004 -> [w7153 w7155]
          tunnel: w7003 -> [w7152 w7154]
          frame False {
          }
          frame True {
            # "command SET SUFFIX"
            n3302 = call-dynamic "Read State Machine.vi"("error in (no error)"=w7154, "Device in"=w7155) -> ("error out"=w7156:errorcluster, "State Machine.lvclass"=w7160:refnum<class "State Machine.lvclass">, "Device out"=w7159:refnum<class "Channel.lvclass">)  [unwired: 7 in]
            n3303 = call-dynamic "Write State.vi"("error in (no error)"=w7156, "State"=300, "State Machine in"=w7160) -> ("error out"=w7157:errorcluster, "State Machine out"=w7161:refnum<class "State Machine.lvclass">)  [unwired: 7 in]
            n3304 = call-dynamic "Write State Machine.vi"("error in (no error)"=w7157, "State Machine.lvclass"=w7161, "Device in"=w7159) -> ("error out"=w7163:errorcluster, "Device out"=w7162:refnum<class "Channel.lvclass">)  [unwired: 7 in]
          }
        }
        n3305 = case shown="True" w6969 {
          tunnel: [w7141 w7145] -> w6993
          tunnel: [w7140 w7144] -> w6992
          tunnel: w6978 -> [w7141 w7143]
          tunnel: w6977 -> [w7140 w7142]
          frame False {
          }
          frame True {
            # "command SET SUFFIX"
            n3306 = call-dynamic "Read State Machine.vi"("error in (no error)"=w7142, "Device in"=w7143) -> ("error out"=w7151:errorcluster, "State Machine.lvclass"=w7147:refnum<class "State Machine.lvclass">, "Device out"=w7148:refnum<class "Channel.lvclass">)  [unwired: 7 in]
            n3307 = call-dynamic "Write State.vi"("error in (no error)"=w7151, "State"=300, "State Machine in"=w7147) -> ("error out"=w7150:errorcluster, "State Machine out"=w7146:refnum<class "State Machine.lvclass">)  [unwired: 7 in]
            n3308 = call-dynamic "Write State Machine.vi"("error in (no error)"=w7150, "State Machine.lvclass"=w7146, "Device in"=w7148) -> ("error out"=w7144:errorcluster, "Device out"=w7145:refnum<class "Channel.lvclass">)  [unwired: 7 in]
          }
        }
        n3309 = call-dynamic "Write Channel.vi"("error in (no error)"=w7070, "Channel.lvclass"=w7071, "Acquisition in"=w7072) -> ("error out"=w7131:errorcluster, "Acquisition out"=w7132:refnum<class "Acquisition.lvclass">)  [unwired: 7 in]
        n3310 = call-dynamic "Write Channel.vi"("error in (no error)"=w7046, "Channel.lvclass"=w7045, "Acquisition in"=w7044) -> ("error out"=w7126:errorcluster, "Acquisition out"=w7127:refnum<class "Acquisition.lvclass">)  [unwired: 7 in]
        n3311 = call-dynamic "Write Channel.vi"("error in (no error)"=w7020, "Channel.lvclass"=w7019, "Acquisition in"=w7018) -> ("error out"=w7115:errorcluster, "Acquisition out"=w7116:refnum<class "Acquisition.lvclass">)  [unwired: 7 in]
        n3312 = call-dynamic "Write Channel.vi"("error in (no error)"=w6992, "Channel.lvclass"=w6993, "Acquisition in"=w6994) -> ("error out"=w7113:errorcluster, "Acquisition out"=w7114:refnum<class "Acquisition.lvclass">)  [unwired: 7 in]
        n3313 = call-dynamic "Write AcquisitionA.vi"("error in (no error)"=w7131, "Acquisition.lvclass"=w7132, "S4ACS_GUI in"=w7133) -> ("error out"=w7121:errorcluster, "S4ACS_GUI out"=w7125:refnum<class "S4GUI.lvclass">)  [unwired: 7 in]
        n3314 = call "Write AcquisitionB.vi"("error in (no error)"=w7126, "Acquisition.lvclass"=w7127, "S4ACS_GUI in"=w7125) -> ("error out"=w7120:errorcluster, "S4ACS_GUI out"=w7124:refnum<class "S4GUI.lvclass">)  [unwired: 7 in]
        n3315 = call-dynamic "Write AcquisitionC.vi"("error in (no error)"=w7115, "Acquisition.lvclass"=w7116, "S4ACS_GUI in"=w7124) -> ("error out"=w7119:errorcluster, "S4ACS_GUI out"=w7123:refnum<class "S4GUI.lvclass">)  [unwired: 7 in]
        n3316 = call-dynamic "Write AcquisitionD.vi"("error in (no error)"=w7113, "Acquisition.lvclass"=w7114, "S4ACS_GUI in"=w7123) -> ("error out"=w7118:errorcluster, "S4ACS_GUI out"=w7122:refnum<class "S4GUI.lvclass">)  [unwired: 7 in]
        n3317 = Merge Errors(w7121, w7120, w7119, w7118) -> (w7117:errorcluster)
        n3318 = call "Write cfg file.vi"("error in (no error)"=w7117, "cfg file"="lastsaved.cfg", "S4ACS_GUI in"=w7122) -> ("error out"=w7129:errorcluster, "S4ACS_GUI out"=w7128:refnum<class "S4GUI.lvclass">)  [unwired: 7 in]
      }
      event "Object_sflat", "Object_dark", "Object_zero", "Object_dflat", "Object_focus", "Object_obj": Value Change {
        n3319 = event-data() -> ("NewVal"=w7212:string)  [unwired: 1 in, 5 out]
        n3320 = stacked-sequence {
          seq-local: [w7242 _ _ _] -> [_ w7306 _ _]
          seq-local: [w7241 _ _ _] -> [_ w7305 _ _]
          seq-local: [_ w7304 _ _] -> [_ _ w7355 _]
          seq-local: [_ w7303 _ _] -> [_ _ w7354 _]
          seq-local: [_ _ w7353 _] -> [_ _ _ w7404]
          seq-local: [_ _ w7352 _] -> [_ _ _ w7403]
          tunnel: w7219 -> [w7254 _ _ _]
          tunnel: w7220 -> [w7253 _ _ _]
          tunnel: [_ _ _ w7402] -> w7214
          tunnel: [_ _ _ w7401] -> w7213
          tunnel: w7218 -> [w7240 w7302 w7351 w7400]
          tunnel: w7217 -> [w7239 w7301 w7337 w7386]
          tunnel: w7215 -> [w7238 w7287 w7336 w7385]
          tunnel: w7212 -> [w7237 w7286 w7335 w7384]
          tunnel: w7216 -> [w7236 w7285 w7334 w7383]
          frame #0 {
            # "observer"
            # "comment"
            # "object"
            # "suffix"
            # "obsType"
            n3321 = call-dynamic "Read AcquisitionA.vi"("error in (no error)"=w7254, "S4ACS_GUI in"=w7253) -> ("error out"=w7252:errorcluster, "Acquisition.lvclass"=w7251:refnum<class "Acquisition.lvclass">, "S4ACS_GUI out"=w7246:refnum<class "S4GUI.lvclass">)  [unwired: 7 in]
            n3322 = call-dynamic "Read Channel.vi"("error in (no error)"=w7252, "Acquisition in"=w7251) -> ("error out"=w7222:errorcluster, "Channel.lvclass"=w7225:refnum<class "Channel.lvclass">, "Acquisition out"=w7245:refnum<class "Acquisition.lvclass">)  [unwired: 7 in]
            n3323 = local read "Filter1"() -> (w7223:u8)
            n3324 = call-dynamic "Write Filter.vi"("error in (no error)"=w7222, "Filter"=w7223, "Channel in"=w7225) -> ("error out"=w7221:errorcluster, "Channel out"=w7224:refnum<class "Channel.lvclass">)  [unwired: 7 in]
            n3325 = call-dynamic "Read Interface.vi"("error in (no error)"=w7221, "Channel in"=w7224) -> ("error out"=w7232:errorcluster, "Interface.lvclass"=w7233:refnum<class "Interface.lvclass">, "Channel out"=w7250:refnum<class "Channel.lvclass">)  [unwired: 7 in]
            n3326 = call-dynamic "Write Suffix.vi"("error in (no error)"=w7232, "Suffix"=w7240, "Interface in"=w7233) -> ("error out"=w7257:errorcluster, "Interface out"=w7249:refnum<class "Interface.lvclass">)  [unwired: 7 in]
            n3327 = call-dynamic "Write ObsType.vi"("error in (no error)"=w7257, "ObsType"=w7238, "Interface in"=w7249) -> ("error out"=w7256:errorcluster, "Interface out"=w7248:refnum<class "Interface.lvclass">)  [unwired: 7 in]
            n3328 = call-dynamic "Write Object.vi"("error in (no error)"=w7256, "Object"=w7237, "Interface in"=w7248) -> ("error out"=w7255:errorcluster, "Interface out"=w7247:refnum<class "Interface.lvclass">)  [unwired: 7 in]
            n3329 = call-dynamic "Write Comments.vi"("error in (no error)"=w7255, "Comments"=w7239, "Interface in"=w7247) -> ("error out"=w7235:errorcluster, "Interface out"=w7234:refnum<class "Interface.lvclass">)  [unwired: 7 in]
            n3330 = call-dynamic "Write Observer.vi"("error in (no error)"=w7235, "Observer"=w7236, "Interface in"=w7234) -> ("error out"=w7230:errorcluster, "Interface out"=w7231:refnum<class "Interface.lvclass">)  [unwired: 7 in]
            n3331 = call-dynamic "Write Interface.vi"("error in (no error)"=w7230, "Interface.lvclass"=w7231, "Channel in"=w7250) -> ("error out"=w7227:errorcluster, "Channel out"=w7229:refnum<class "Channel.lvclass">)  [unwired: 7 in]
            n3332 = disable-structure shown="Enabled" {
              disable-tunnel: w7229 -> [w7267 w7269]
              disable-tunnel: [w7265 w7269] -> w7228
              disable-tunnel: w7227 -> [w7264 w7268]
              disable-tunnel: [w7259 w7268] -> w7226
              frame Disabled {
                n3333 = call-dynamic "Read State Machine.vi"("error in (no error)"=w7264, "Device in"=w7267) -> ("error out"=w7263:errorcluster, "State Machine.lvclass"=w7261:refnum<class "State Machine.lvclass">, "Device out"=w7266:refnum<class "Channel.lvclass">)  [unwired: 7 in]
                n3334 = call "Next State.vi"("error in (no error)"=w7263, "New_State"=12, "State Machine in"=w7261) -> ("error out"=w7262:errorcluster, "State Machine out"=w7260:refnum<class "State Machine.lvclass">)  [unwired: 7 in]
                n3335 = call-dynamic "Write State Machine.vi"("error in (no error)"=w7262, "State Machine.lvclass"=w7260, "Device in"=w7266) -> ("error out"=w7259:errorcluster, "Device out"=w7265:refnum<class "Channel.lvclass">)  [unwired: 7 in]
              }
              frame Enabled {
              }
            }
            n3336 = call-dynamic "Write Channel.vi"("error in (no error)"=w7226, "Channel.lvclass"=w7228, "Acquisition in"=w7245) -> ("error out"=w7243:errorcluster, "Acquisition out"=w7244:refnum<class "Acquisition.lvclass">)  [unwired: 7 in]
            n3337 = call-dynamic "Write AcquisitionA.vi"("error in (no error)"=w7243, "Acquisition.lvclass"=w7244, "S4ACS_GUI in"=w7246) -> ("error out"=w7241:errorcluster, "S4ACS_GUI out"=w7242:refnum<class "S4GUI.lvclass">)  [unwired: 7 in]
          }
          frame #1 {
            # "object"
            # "suffix"
            # "obsType"
            n3338 = call "Read AcquisitionB.vi"("error in (no error)"=w7305, "S4ACS_GUI in"=w7306) -> ("error out"=w7291:errorcluster, "Acquisition.lvclass"=w7292:refnum<class "Acquisition.lvclass">, "S4ACS_GUI out"=w7297:refnum<class "S4GUI.lvclass">)  [unwired: 7 in]
            n3339 = call-dynamic "Read Channel.vi"("error in (no error)"=w7291, "Acquisition in"=w7292) -> ("error out"=w7271:errorcluster, "Channel.lvclass"=w7273:refnum<class "Channel.lvclass">, "Acquisition out"=w7298:refnum<class "Acquisition.lvclass">)  [unwired: 7 in]
            n3340 = local read "Filter2"() -> (w7274:u8)
            n3341 = call-dynamic "Write Filter.vi"("error in (no error)"=w7271, "Filter"=w7274, "Channel in"=w7273) -> ("error out"=w7270:errorcluster, "Channel out"=w7272:refnum<class "Channel.lvclass">)  [unwired: 7 in]
            n3342 = call-dynamic "Read Interface.vi"("error in (no error)"=w7270, "Channel in"=w7272) -> ("error out"=w7279:errorcluster, "Interface.lvclass"=w7280:refnum<class "Interface.lvclass">, "Channel out"=w7293:refnum<class "Channel.lvclass">)  [unwired: 7 in]
            n3343 = call-dynamic "Write Suffix.vi"("error in (no error)"=w7279, "Suffix"=w7302, "Interface in"=w7280) -> ("error out"=w7288:errorcluster, "Interface out"=w7294:refnum<class "Interface.lvclass">)  [unwired: 7 in]
            n3344 = call-dynamic "Write ObsType.vi"("error in (no error)"=w7288, "ObsType"=w7287, "Interface in"=w7294) -> ("error out"=w7289:errorcluster, "Interface out"=w7295:refnum<class "Interface.lvclass">)  [unwired: 7 in]
            n3345 = call-dynamic "Write Object.vi"("error in (no error)"=w7289, "Object"=w7286, "Interface in"=w7295) -> ("error out"=w7290:errorcluster, "Interface out"=w7296:refnum<class "Interface.lvclass">)  [unwired: 7 in]
            n3346 = call-dynamic "Write Comments.vi"("error in (no error)"=w7290, "Comments"=w7301, "Interface in"=w7296) -> ("error out"=w7282:errorcluster, "Interface out"=w7281:refnum<class "Interface.lvclass">)  [unwired: 7 in]
            n3347 = call-dynamic "Write Observer.vi"("error in (no error)"=w7282, "Observer"=w7285, "Interface in"=w7281) -> ("error out"=w7283:errorcluster, "Interface out"=w7284:refnum<class "Interface.lvclass">)  [unwired: 7 in]
            n3348 = call-dynamic "Write Interface.vi"("error in (no error)"=w7283, "Interface.lvclass"=w7284, "Channel in"=w7293) -> ("error out"=w7277:errorcluster, "Channel out"=w7278:refnum<class "Channel.lvclass">)  [unwired: 7 in]
            n3349 = disable-structure shown="Enabled" {
              disable-tunnel: w7278 -> [w7311 w7318]
              disable-tunnel: w7277 -> [w7310 w7317]
              disable-tunnel: [w7308 w7318] -> w7276
              disable-tunnel: [w7307 w7317] -> w7275
              frame Disabled {
                n3350 = call-dynamic "Read State Machine.vi"("error in (no error)"=w7310, "Device in"=w7311) -> ("error out"=w7316:errorcluster, "State Machine.lvclass"=w7314:refnum<class "State Machine.lvclass">, "Device out"=w7309:refnum<class "Channel.lvclass">)  [unwired: 7 in]
                n3351 = call "Next State.vi"("error in (no error)"=w7316, "New_State"=12, "State Machine in"=w7314) -> ("error out"=w7315:errorcluster, "State Machine out"=w7313:refnum<class "State Machine.lvclass">)  [unwired: 7 in]
                n3352 = call-dynamic "Write State Machine.vi"("error in (no error)"=w7315, "State Machine.lvclass"=w7313, "Device in"=w7309) -> ("error out"=w7307:errorcluster, "Device out"=w7308:refnum<class "Channel.lvclass">)  [unwired: 7 in]
              }
              frame Enabled {
              }
            }
            n3353 = call-dynamic "Write Channel.vi"("error in (no error)"=w7275, "Channel.lvclass"=w7276, "Acquisition in"=w7298) -> ("error out"=w7300:errorcluster, "Acquisition out"=w7299:refnum<class "Acquisition.lvclass">)  [unwired: 7 in]
